vi "Generate Registration Trace.vi"(9 "Event Name":string, 10 "Registrant Address":refnum<class "Message Enqueuer.lvclass">, 11 "Event Source Address":refnum<class "Message Enqueuer.lvclass">) -> ()   [LabVIEW 2016]
uses:
  <vilib>/ActorFramework/Message Enqueuer/Message Enqueuer.lvclass
  <resource>/AFDebug/Registration Mode.ctl
  <resource>/AFDebug/AF Debug.lvlib
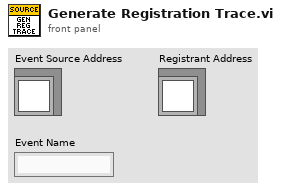
[diagram p1: front panel]
types:
  T1 = typedef "AF Debug.lvlib/Registration Mode.ctl" = enum16{"Register Actor", "Get ID", "Get Enqueuer", "Deregister Actor"}
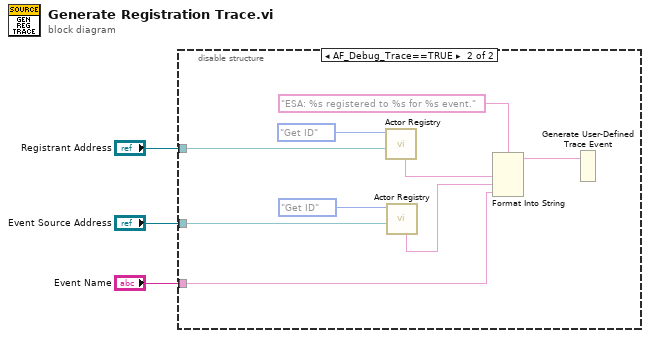
[diagram p0: block diagram]
diagram:
  n1 = disable-structure shown="AF_Debug_Trace==TRUE" {
    disable-tunnel: "Event Source Address" -> [_ w10]
    disable-tunnel: "Registrant Address" -> [_ w9]
    disable-tunnel: "Event Name" -> [_ w4]
    frame condition #0 (active) {
    }
    frame condition #1 {
      n2 = call <resource>:"Actor Registry.vi"("Actor Enqueuer"=w9, "Action"=Registration_Mode."Get ID") -> ("Actor Alias out"=w6:string)  [unwired: 5 in, 4 out]
      n3 = call <resource>:"Actor Registry.vi"("Actor Enqueuer"=w10, "Action"=Registration_Mode."Get ID") -> ("Actor Alias out"=w5:string)  [unwired: 5 in, 4 out]
      n4 = Format Into String(format string="ESA: %s registered to %s for %s event.", w6, w5, w4) -> (resulting string=w8:string)  [unwired: 2 in, 1 out]
      n5 = Generate User-Defined Trace Event(2:w8) -> ()  [unwired: 1 in]
    }
  }
